vi "CompileParsePulseSeq.vi"(11 "PulseSeqIn":string) -> (0 "error out":errorcluster, 1 "Params":T2, 2 "RFPulseList":string, 3 "PulseList":T1[](array[typedef]))   [LabVIEW 2019]
uses:
  Params.ctl
  SinglePulse.ctl
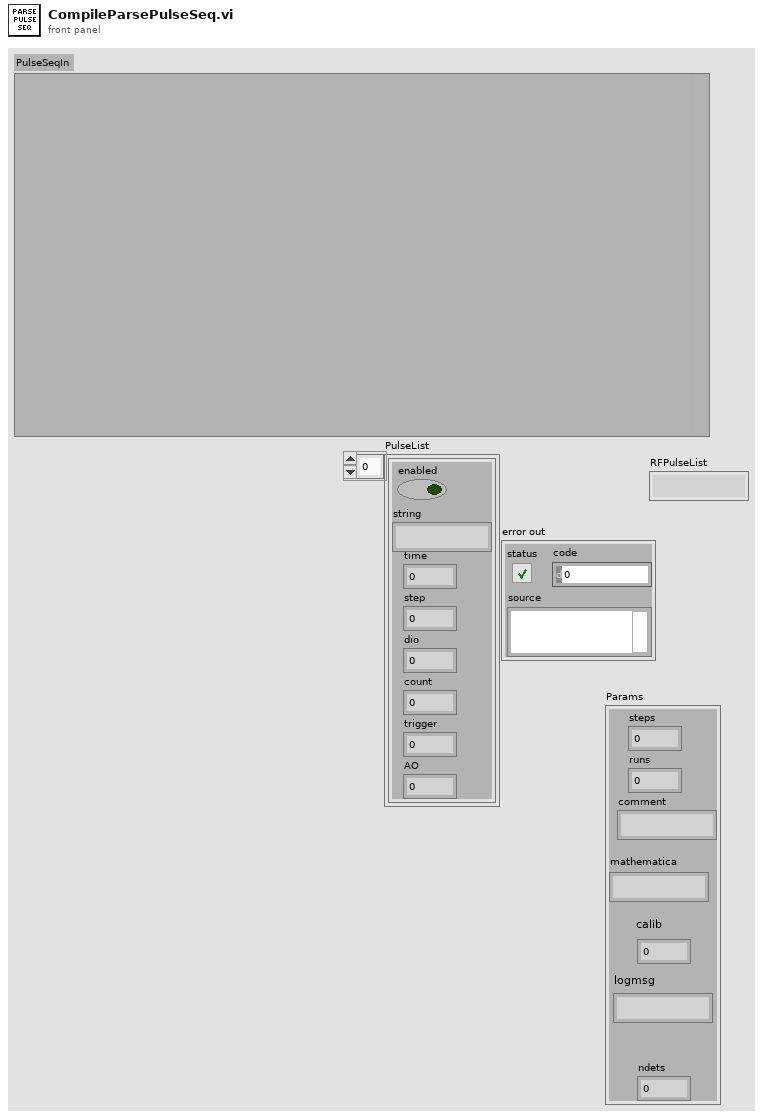
[diagram p1: front panel]
types:
  T1 = typedef "SinglePulse.ctl" = cluster{"enabled":bool, "string":string, "time":dbl, "step":dbl, "dio":dbl, "count":dbl, "trigger":dbl, "AO":dbl}
  T2 = typedef "Params.ctl" = cluster{"steps":i16, "runs":i16, "comment":string, "mathematica":string, "calib":i8, "logmsg":string, "ndets":i16}
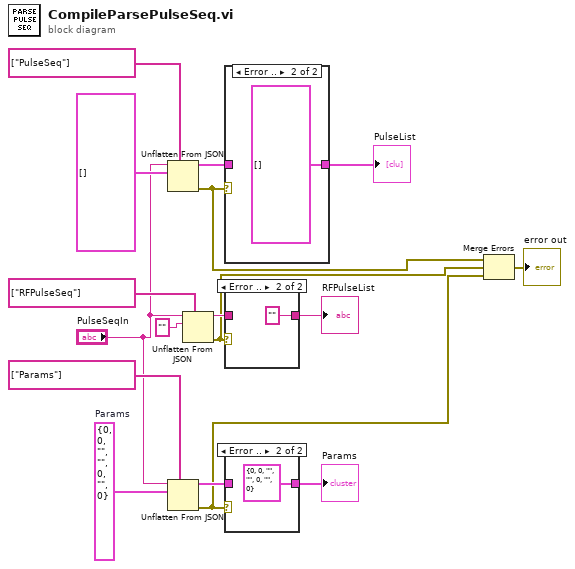
[diagram p0: block diagram]
diagram:
  w11 = T2 {"steps"=0, "runs"=0, "comment"="", "mathematica"="", "calib"=0, "logmsg"="", "ndets"=0}  # Params
  n1 = Unflatten From JSON(path=string[] ["PulseSeq"], JSON string="PulseSeqIn", type and defaults=T1[] []) -> (value=w6:T1[], error out=w4:errorcluster)  [unwired: 4 in]
  n2 = Unflatten From JSON(path=string[] ["Params"], JSON string="PulseSeqIn", type and defaults=w11) -> (value=w8:T2, error out=w2:errorcluster)  [unwired: 4 in]
  n3 = Unflatten From JSON(path=string[] ["RFPulseSeq"], JSON string="PulseSeqIn", type and defaults="") -> (value=w10:string, error out=w3:errorcluster)  [unwired: 4 in]
  n4 = case shown="Error .." w4 {
    tunnel: w6 -> [w18 _]
    tunnel: [w18 T1[] []] -> w5
    frame No Error {
    }
    frame Error {
    }
  }
  "PulseList" <- w5
  n5 = case shown="Error .." w3 {
    tunnel: w10 -> [w20 _]
    tunnel: [w20 ""] -> w9
    frame No Error {
    }
    frame Error {
    }
  }
  "RFPulseList" <- w9
  n6 = case shown="Error .." w2 {
    tunnel: w8 -> [w22 _]
    tunnel: [w22 T2 {"steps"=0, "runs"=0, "comment"="", "mathematica"="", "calib"=0, "logmsg"="", "ndets"=0} ("Params")] -> w7
    frame No Error {
    }
    frame Error {
    }
  }
  "Params" <- w7
  n7 = Merge Errors(w4, w3, w2) -> (→"error out":errorcluster)
